vi "Ctor.vi"(4 "Timeout ms":i32, 8 "error in (no error)":errorcluster, 9 "Server Stream":bool, 10 "Command Queue":refnum<queue>, 11 "TCP Connection":refnum<k5>) -> (0 "error out":errorcluster, 3 "WebsocketStream out":refnum<class "WebsocketStream.lvclass">)   [LabVIEW 2020, in "Stream-Websocket.lvlib" / "WebsocketStream.lvclass"]
uses:
  WebsocketStream.lvclass
  Client Command.ctl
  Ref Data.ctl
  WebsocketStream.lvclass/WebsocketStream.ctl
  Stream-Websocket.lvlib
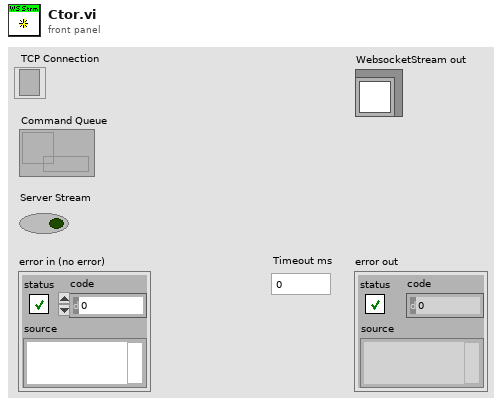
[diagram p1: front panel]
types:
  T1 = typedef "Stream-Websocket.lvlib/WebsocketStream.lvclass/Ref Data.ctl" = cluster{"Command Queue":refnum<queue>, "Closing":bool}
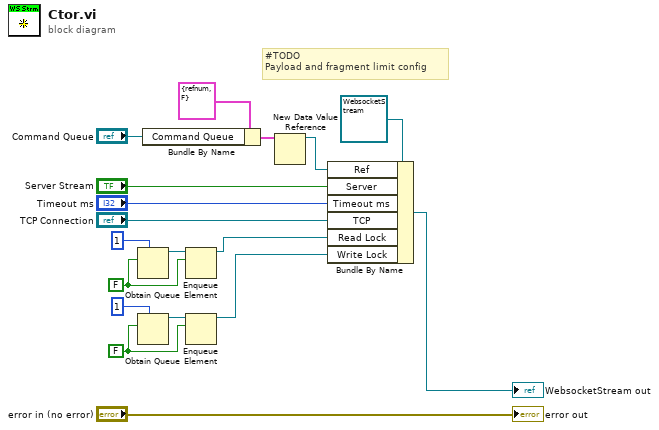
[diagram p0: block diagram]
diagram:
  w3 = FALSE
  w8 = FALSE
  # "#TODO\nPayload and fragment limit config"
  n1 = Obtain Queue(max queue size (-1, unlimited)=1, element data type=w8) -> (queue out=w9:refnum<queue>)  [unwired: 3 in, 2 out]
  n2 = Obtain Queue(max queue size (-1, unlimited)=1, element data type=w3) -> (queue out=w2:refnum<queue>)  [unwired: 3 in, 2 out]
  n3 = Bundle By Name(cluster=T1 {"Command Queue"=refnum, "Closing"=FALSE} ("Ref Data"), "Command Queue"="Command Queue") -> (w12:T1)
  n4 = Enqueue Element(queue=w9, element=w8) -> (queue out=w6:refnum<queue>)  [unwired: 2 in, 2 out]
  n5 = Enqueue Element(queue=w2, element=w3) -> (queue out=w1:refnum<queue>)  [unwired: 2 in, 2 out]
  n6 = New Data Value Reference(data value=w12) -> (data value reference=w11:refnum<data-value>)  [unwired: 1 in, 1 out]
  n7 = Bundle By Name(cluster=refnum<class "WebsocketStream.lvclass"> refnum ("WebsocketStream in"), "Ref"=w11, "Server"="Server Stream", "Timeout ms"="Timeout ms", "TCP"="TCP Connection", "Read Lock"=w6, "Write Lock"=w1) -> (→"WebsocketStream out":refnum<class "WebsocketStream.lvclass">)
  "error out" <- "error in (no error)"
